vi "Check Help.vi"(8 "error in (no error)":errorcluster, 11 "LV Argument Parser in":refnum<class "LV Argument Parser.lvclass">) -> (0 "error out":errorcluster, 2 "Output":string, 3 "LV Argument Parser out":refnum<class "LV Argument Parser.lvclass">)   [LabVIEW 2023, in "LV ArgParse.lvlib" / "LV Argument Parser.lvclass"]
uses:
  LV Argument Parser.lvclass
  LV Argument Parser.lvclass/LV Argument Parser.ctl
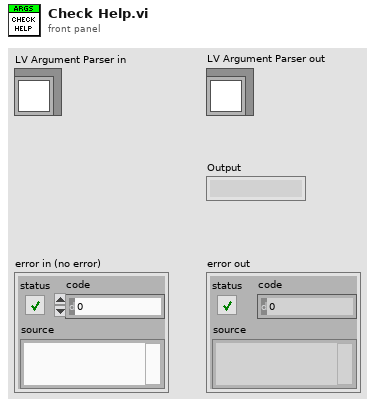
[diagram p1: front panel]
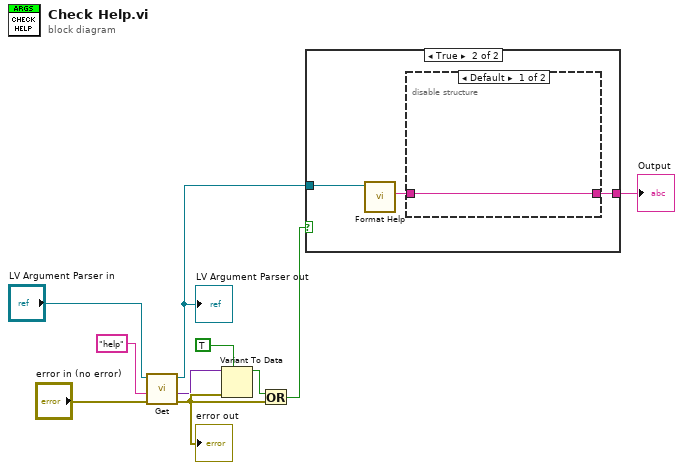
[diagram p0: block diagram]
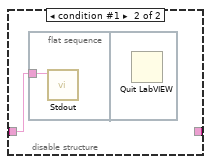
[diagram p3: hidden frame]
diagram:
  n1 = call "Get.vi"("error in (no error)"="error in (no error)", "Name"="help", "LV Argument Parser in"="LV Argument Parser in") -> ("error out"=w7:errorcluster, "element"=w6:variant, "LV Argument Parser out"=w10:refnum<class "LV Argument Parser.lvclass">)  [unwired: 5 in, 1 out]
  "error out" <- w7
  "LV Argument Parser out" <- w10
  n2 = Variant To Data(error in=w7, type=TRUE ("Optional"), Variant=w6) -> (data=w9:bool)  [unwired: 1 out]
  n3 = Or(x=w9, y=w7) -> (x .or. y?=w5:bool)
  n4 = case shown="True" w5 {
    tunnel: w10 -> [_ w12]
    tunnel: [_ w11] -> w2
    frame False {
    }
    frame True {
      n5 = call "Format Help.vi"("LV Argument Parser in"=w12) -> ("String"=w13:string)  [unwired: 8 in, 2 out]
      n6 = disable-structure shown="Default" {
        disable-tunnel: w13 -> [w14 w15]
        disable-tunnel: [w14 _] -> w11
        frame condition #0 (active) {
        }
        frame condition #1 {
          n7 = flat-sequence {
            tunnel: w15 -> [w16]
            frame #0 {
              n8 = call "Stdout.vi"("text"=w16) -> ()  [unwired: 10 in, 1 out]
            }
            frame #1 {
              n9 = Quit LabVIEW() -> ()  [unwired: 1 in]
            }
          }
        }
      }
    }
  }
  "Output" <- w2
